vi "Wash Needle.vi"(8 "error in (no error)":errorcluster, 11 "Autosampler in":refnum<class "Autosampler.lvclass">) -> (0 "error out":errorcluster, 3 "Autosampler out":refnum<class "Autosampler.lvclass">)   [LabVIEW 2023, in "Autosampler.lvlib" / "Autosampler.lvclass"]
uses:
  Autosampler.lvclass
  Autosampler.lvclass/Autosampler.ctl
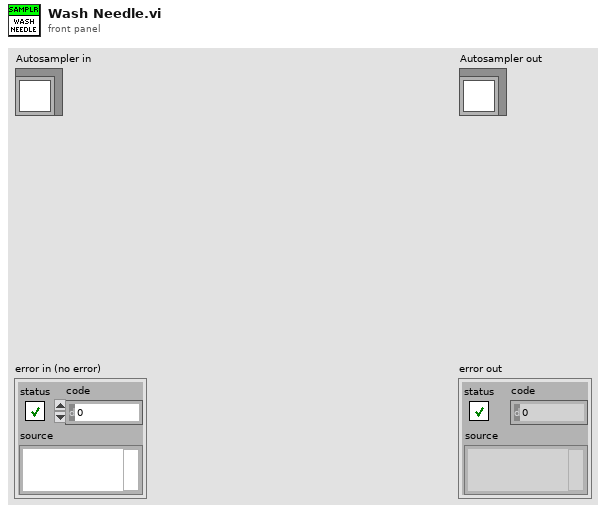
[diagram p1: front panel]
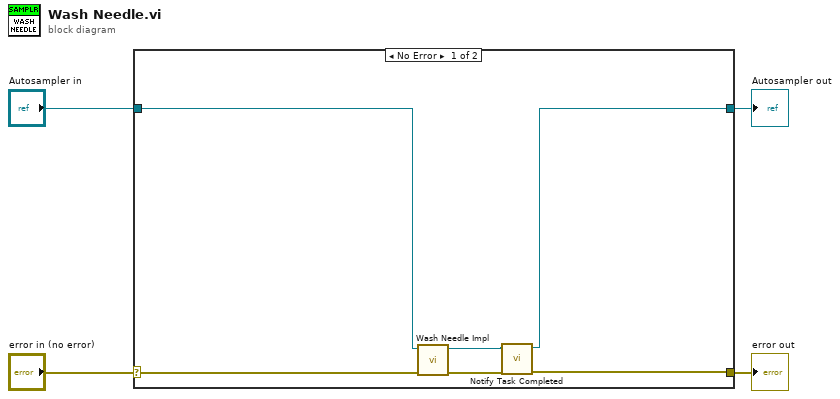
[diagram p0: block diagram]
diagram:
  n1 = case shown="No Error" "error in (no error)" {
    selector: "error in (no error)" -> [w10 w12]
    tunnel: [w7 w12] -> w3
    tunnel: [w5 w11] -> w1
    tunnel: "Autosampler in" -> [w9 w11]
    frame No Error {
      n2 = call-dynamic "Wash Needle Impl.vi"("error in (no error)"=w10, "Autosampler in"=w9) -> ("error out"=w8:errorcluster, "Autosampler out"=w6:refnum<class "Autosampler.lvclass">)  [unwired: 8 in]
      n3 = call-dynamic "Notify Task Completed.vi"("error in (no error)"=w8, "Device in"=w6) -> ("error out"=w7:errorcluster, "Device out"=w5:refnum<class "Autosampler.lvclass">)  [unwired: 8 in]
    }
    frame Error {
    }
  }
  "error out" <- w3
  "Autosampler out" <- w1
